vi "HAL camera calculate binning - SubVI.vi"(11 "Camera Parameters (important)":T1={"Exposure Time (sec)"=0.0, "EM CCD Gain"=230, "Readout Settings"={"Acquisition Mode"=enum."(do not use)", "Pixel Rate"=enum."EM CCD 10 Mhz 14 bits", "High Capacity?"=FALSE, "V Shift Speed (us/row)"=enum."0.4 (not reccommended)", "V Shift Amplitude"=enum."normal", "Preamp Gain"=enum."2.6", "Trigger Mode"=0}, "Image Size"={"H Bin"=1, "V Bin"=1, "Left"=1, "Top"=1, "Right"=512, "Bottom"=512}, "Shutter"=0} {"Shutter" items=["Auto", "Stay Open", "Always Closed"]; "Readout Settings"."Trigger Mode" items=["Internal", "External"]; "EM CCD Gain" scale=0.01..255.0; "Exposure Time (sec)" scale=0.001..10.0 scale format="%#_1g"}) -> (2 "V Bin":i32, 3 "H Bin":i32)   [LabVIEW 2014]
uses:
  HAL camera parameters important 1 - SubVI.ctl
  ixon readout settings - SubVI.ctl
  andor acquisition mode.ctl
  image size - SubVI.ctl
panel:
  # "Camera: Andor iXon"
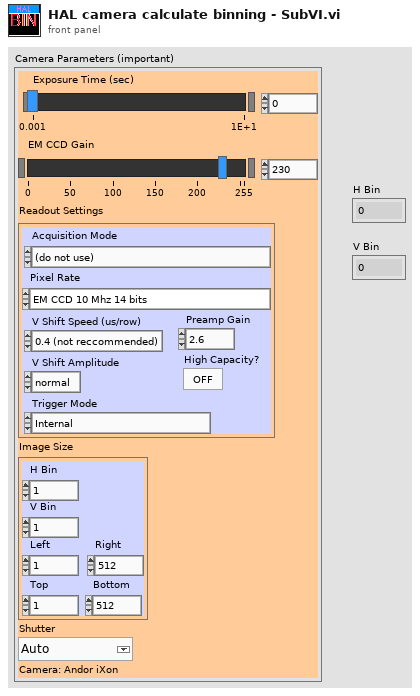
[diagram p1: front panel]
types:
  T1 = typedef "HAL camera parameters important 1 - SubVI.ctl" = cluster{"Exposure Time (sec)":sgl, "EM CCD Gain":u8, "Readout Settings":T2, "Image Size":T4, "Shutter":i32}
  T2 = typedef "ixon readout settings - SubVI.ctl" = cluster{"Acquisition Mode":T3, "Pixel Rate":enum16{"EM CCD 10 Mhz 14 bits", "EM CCD 5 Mhz 14 bits", "EM CCD 3 Mhz 14 bits", "EM CCD 1 Mhz 16 bits", "Standard CCD 3 Mhz 14 bits", "Standard CCD 1 Mhz 16 bits"}, "High Capacity?":bool, "V Shift Speed (us/row)":enum16{"0.4 (not reccommended)", "0.6  (not reccommended)", "1.0  (not reccommended)", "1.8  (not reccommended)", "3.4  (not reccommended)", "6.6", "13.0"}, "V Shift Amplitude":enum16{"normal", "+1", "+2", "+3", "+4"}, "Preamp Gain":enum16{"1.0", "2.6"}, "Trigger Mode":u32}
  T3 = typedef "andor acquisition mode.ctl" = enum16{"(do not use)", "Single Scan", "Accumulate", "Kinetics", "Fast Kinetics", "Kinetics Run till Abort", "Frame Transfer", "Frame Transfer Run till Abort", "(do not use) ", "Time Delayed Integration"}
  T4 = typedef "image size - SubVI.ctl" = cluster{"H Bin":i32, "V Bin":i32, "Left":i32, "Top":i32, "Right":i32, "Bottom":i32}
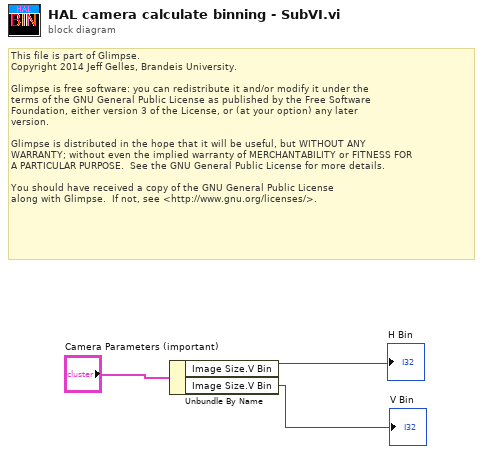
[diagram p0: block diagram]
diagram:
  # "This file is part of Glimpse. \nCopyright 2014 Jeff Gelles, Brandeis University.    \n\nGlimpse is free software: you can redistribute it and/or modify it under the \nterms of the GNU General Public License as published by the Free Software \nFoundation, either version 3 of the License, or (at your option) any later \nversion.\n\nGlimpse is distributed in the hope that it will be useful, but WITHOUT ANY \nWARRANTY; without even the implied warranty of MERCHANTABILITY or FITNESS FOR \nA PARTICULAR PURPOSE.  See the GNU General Public License for more details.\n\nYou should have received a copy of the GNU General Public License\nalong with Glimpse.  If not, see <http://www.gnu.org/licenses/>."
  n1 = Unbundle By Name("Camera Parameters (important)") -> ("Image Size.V Bin"=→"H Bin":i32, "Image Size.V Bin"=→"V Bin":i32)
